vi "Write Iterator Enqueuer.vi"(8 "error in (no error)":errorcluster, 10 "Actor Framework:Message Enqueuer":refnum<class "Message Enqueuer.lvclass">, 11 "Request Iteration Notification Msg in":refnum<class "Request Iteration Notification Msg.lvclass">) -> (0 "error out":errorcluster, 3 "Request Iteration Notification Msg out":refnum<class "Request Iteration Notification Msg.lvclass">)   [LabVIEW 2023, in "Iterator Actor.lvlib" / "Request Iteration Notification Msg.lvclass"]
uses:
  Request Iteration Notification Msg.lvclass
  <vilib>/ActorFramework/Message Enqueuer/Message Enqueuer.lvclass
  Request Iteration Notification Msg.lvclass/Request Iteration Notification Msg.ctl
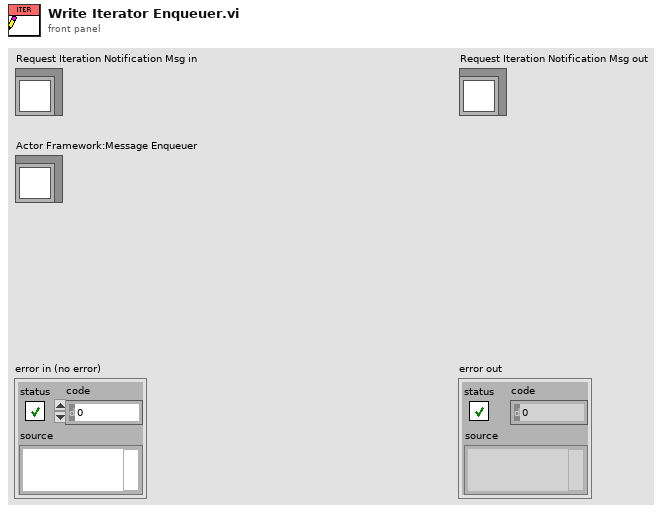
[diagram p1: front panel]
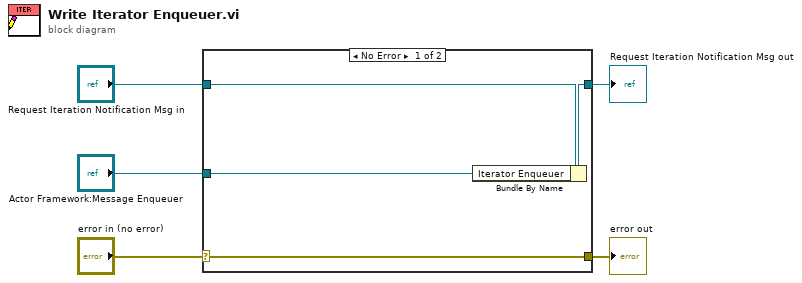
[diagram p0: block diagram]
diagram:
  n1 = case shown="No Error" "error in (no error)" {
    selector: "error in (no error)" -> [w9 w10]
    tunnel: [w9 w10] -> w4
    tunnel: [w7 w11] -> w2
    tunnel: "Request Iteration Notification Msg in" -> [w8 w11]
    tunnel: "Actor Framework:Message Enqueuer" -> [w6 _]
    frame No Error {
      n2 = Bundle By Name(cluster=w8, "Iterator Enqueuer"=w6) -> (w7:refnum<class "Request Iteration Notification Msg.lvclass">)
    }
    frame Error {
    }
  }
  "error out" <- w4
  "Request Iteration Notification Msg out" <- w2
